vi "StartFeedback.vi"(0 "State":i32, 5 "error in":T1) -> (14 "State out":i32, 19 "error out":T1)   [LabVIEW 2016]
doc: "Starts (state = 1) or stops (state = 0) the z control."
uses:
  Controls/Error_Out.ctl
  Files_ASC500/DLL/ASC500_RemoteControlV27.dll
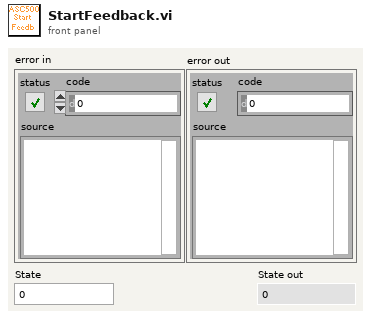
[diagram p1: front panel]
types:
  T1 = typedef "Error_Out.ctl" = errorcluster
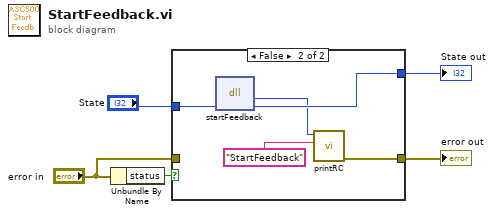
[diagram p0: block diagram]
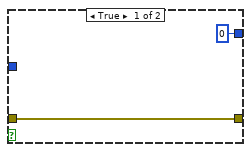
[diagram p2: hidden frame]
diagram:
  n1 = Unbundle By Name("error in") -> ("status"=w5:bool)
  n2 = case shown="False" w5 {
    tunnel: [w6 w10] -> w4
    tunnel: [0 ("State") w12] -> w3
    tunnel: "State" -> [_ w11]
    tunnel: "error in" -> [w6 _]
    frame True {
    }
    frame False {
      n3 = dll-call lib="G:/SCMOperations/Share/ELE/Produkt Information/ASC500/04 Remote Control/02 development versions/2018Nov06/Files_ASC500/DLL/ASC500_RemoteControlV27.dll" fn="startFeedback"("State"=w11) -> ("return type"=w9:i32, "State"=w12:i32)  [unwired: 3 in, 2 out]
      n4 = call "printRC.vi"("additional information"="StartFeedback", "RC"=w9) -> ("error out"=w10:T1)  [unwired: 9 in]
    }
  }
  "error out" <- w4
  "State out" <- w3
